vi "复数比较器.vi"(7 "比较模式":enum16{"≠", "＝", "＞", "≥", "＜", "≤"}(ring), 9 "方式":enum16{"按实部", "按虚部", "按幅值", "按相位"}(ring), 10 "c+di":cdb, 11 "a+bi":cdb) -> (3 "结果":bool)   [LabVIEW 2011]
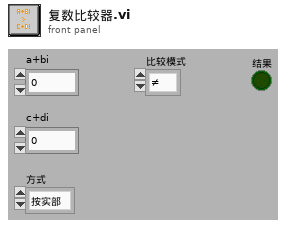
[diagram p1: front panel]
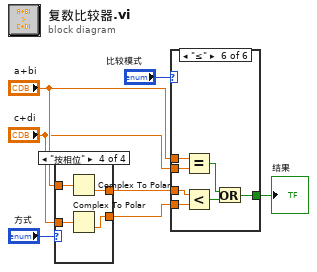
[diagram p0: block diagram]
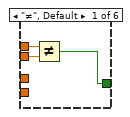
[diagram p2: hidden frame]
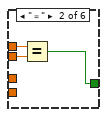
[diagram p3: hidden frame]
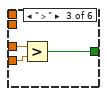
[diagram p4: hidden frame]
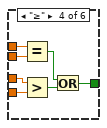
[diagram p5: hidden frame]
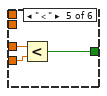
[diagram p6: hidden frame]
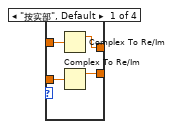
[diagram p7: hidden frame]
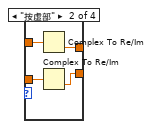
[diagram p8: hidden frame]
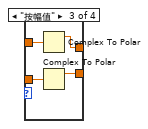
[diagram p9: hidden frame]
diagram:
  n1 = case shown="\"按相位\"" "方式" {
    tunnel: "c+di" -> [w10 w13 w17 w21]
    tunnel: "a+bi" -> [w11 w15 w19 w23]
    tunnel: [w9 w14 w18 w22] -> w2
    tunnel: [w8 w12 w16 w20] -> w1
    frame "按实部", Default {
      n2 = Complex To Re/Im(x + iy=w11) -> (x=w9:dbl)  [unwired: 1 out]
      n3 = Complex To Re/Im(x + iy=w10) -> (x=w8:dbl)  [unwired: 1 out]
    }
    frame "按虚部" {
      n4 = Complex To Re/Im(x + iy=w15) -> (y=w14:dbl)  [unwired: 1 out]
      n5 = Complex To Re/Im(x + iy=w13) -> (y=w12:dbl)  [unwired: 1 out]
    }
    frame "按幅值" {
      n6 = Complex To Polar(r * e^(i*theta)=w19) -> (r=w18:dbl)  [unwired: 1 out]
      n7 = Complex To Polar(r * e^(i*theta)=w17) -> (r=w16:dbl)  [unwired: 1 out]
    }
    frame "按相位" {
      n8 = Complex To Polar(r * e^(i*theta)=w23) -> (theta=w22:dbl)  [unwired: 1 out]
      n9 = Complex To Polar(r * e^(i*theta)=w21) -> (theta=w20:dbl)  [unwired: 1 out]
    }
  }
  n10 = case shown="\"≤\"" "比较模式" {
    tunnel: "a+bi" -> [w26 w29 _ w39 _ w47]
    tunnel: "c+di" -> [w25 w28 _ w38 _ w46]
    tunnel: [w24 w27 w30 w33 w40 w43] -> w3
    tunnel: w2 -> [_ _ w32 w37 w42 w49]
    tunnel: w1 -> [_ _ w31 w36 w41 w48]
    frame "≠", Default {
      n11 = Not Equal?(x=w26, y=w25) -> (x != y?=w24:bool)
    }
    frame "＝" {
      n12 = Equal?(x=w29, y=w28) -> (x = y?=w27:bool)
    }
    frame "＞" {
      n13 = Greater?(x=w32, y=w31) -> (0:w30:bool)
    }
    frame "≥" {
      n14 = Equal?(x=w39, y=w38) -> (x = y?=w34:bool)
      n15 = Greater?(x=w37, y=w36) -> (0:w35:bool)
      n16 = Or(x=w34, y=w35) -> (x .or. y?=w33:bool)
    }
    frame "＜" {
      n17 = Less?(x=w42, y=w41) -> (x < y?=w40:bool)
    }
    frame "≤" {
      n18 = Equal?(x=w47, y=w46) -> (x = y?=w45:bool)
      n19 = Less?(x=w49, y=w48) -> (x < y?=w44:bool)
      n20 = Or(x=w45, y=w44) -> (x .or. y?=w43:bool)
    }
  }
  "结果" <- w3
